vi "termination_condition.vi"(9 "q(0)":dbl[](array[numeric]), 10 "sigma":dbl, 11 "q(i)":dbl[](array[numeric])) -> (3 "Y/N":bool)   [LabVIEW 2022 SP3]
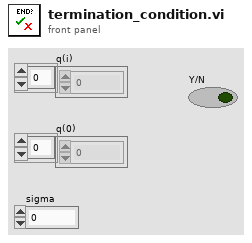
[diagram p1: front panel]
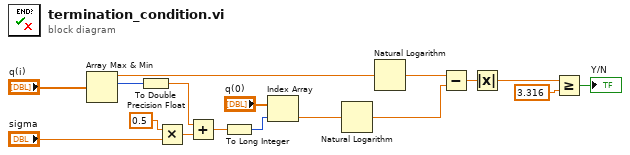
[diagram p0: block diagram]
diagram:
  n1 = Array Max & Min(array="q(i)") -> (max value=w4:dbl, max index (indices)=w6:i32)  [unwired: 2 out]
  n2 = To Double Precision Float(number=w6) -> (double precision float=w5:dbl)
  n3 = Multiply(x=0.5, y="sigma") -> (x*y=w9:dbl)
  n4 = Add(x=w5, y=w9) -> (x+y=w8:dbl)
  n5 = To Long Integer(number=w8) -> (32bit integer=w7:i32)
  n6 = Index Array(array="q(0)", index=w7) -> (element=w1:dbl)
  n7 = Natural Logarithm(1:w1) -> (0:w2:dbl)
  n8 = Natural Logarithm(1:w4) -> (0:w3:dbl)
  n9 = Subtract(x=w3, y=w2) -> (x-y=w11:dbl)
  n10 = Absolute Value(x=w11) -> (abs(x)=w10:dbl)
  n11 = Greater Or Equal?(x=w10, y=3.316) -> (x >= y?=→"Y/N":bool)
